vi "Renishaw-XL80_Close.vi"(8 "error in (no error)":errorcluster, 11 "Renishaw-XL80_EMU in":refnum<class "Renishaw-XL80_EMU.lvclass">) -> (0 "error out":errorcluster, 3 "Renishaw-XL80_EMU out":refnum<class "Renishaw-XL80_EMU.lvclass">)   [LabVIEW 2024, in "Renishaw-XL80_EMU.lvclass"]
doc: "This method disconnects a client from a DX10.\n\nDefinition\nHRESULTDisconnect();\nParameters\nNone\n\n\nComments\nThis method must be called before the client exits. Failing to call this method will at best lead to a reference leak and at worst can mean that the DX10 remains unavailable to other clients.\n\nA similar effect may occur if the client crashes before calling this method. In both cases restarting DX10Server.exe is the only way to recover.\n\nThis method will normally return with an HRESULT of S_OK unless there is an unexpected error. \n\nSee Also"
uses:
  Renishaw-XL80_EMU.lvclass
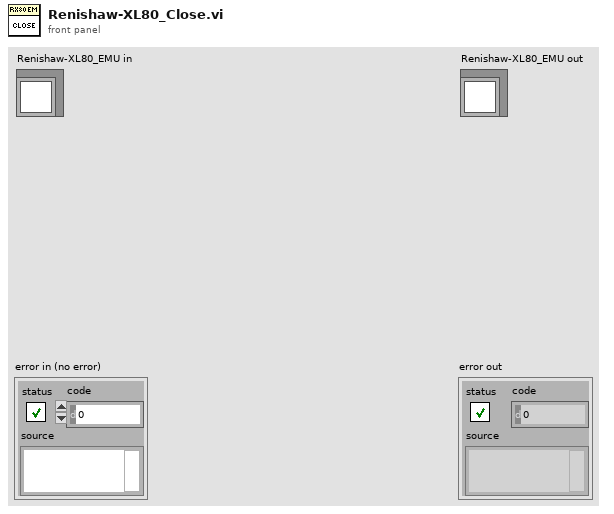
[diagram p1: front panel]
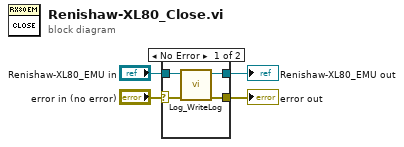
[diagram p0: block diagram]
diagram:
  n1 = case shown="No Error" "error in (no error)" {
    selector: "error in (no error)" -> [w6 w9]
    tunnel: "Renishaw-XL80_EMU in" -> [w8 w10]
    tunnel: [w7 w10] -> w1
    tunnel: [w5 w9] -> w2
    frame No Error {
      n2 = call-dynamic "Log_WriteLog.vi"("error in (no error)"=w6, "Log in"=w8) -> ("error out"=w5:errorcluster, "Log out"=w7:refnum<class "Renishaw-XL80_EMU.lvclass">)  [unwired: 8 in]
    }
    frame Error {
    }
  }
  "error out" <- w2
  "Renishaw-XL80_EMU out" <- w1
